vi "Drive Distance and Speed.vi"(4 "Minimum Speed To ramp to":dbl, 6 "Distance to Start Slowing Down At":dbl, 8 "Wanted Distance Right":dbl, 9 "Wanted Distance Left":dbl, 10 "Wanted Speed Right":dbl, 11 "Wanted Speed Left":dbl) -> (0 "Finished Driving":bool, 1 "Right Output Speed":dbl, 2 "Left Output Speed":dbl)   [LabVIEW 2016]
uses:
  Framework/Robot Global Data.vi
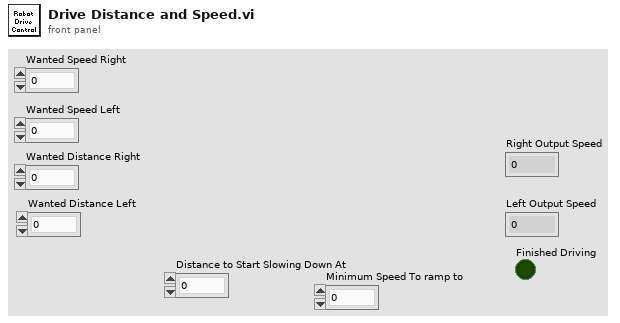
[diagram p1: front panel]
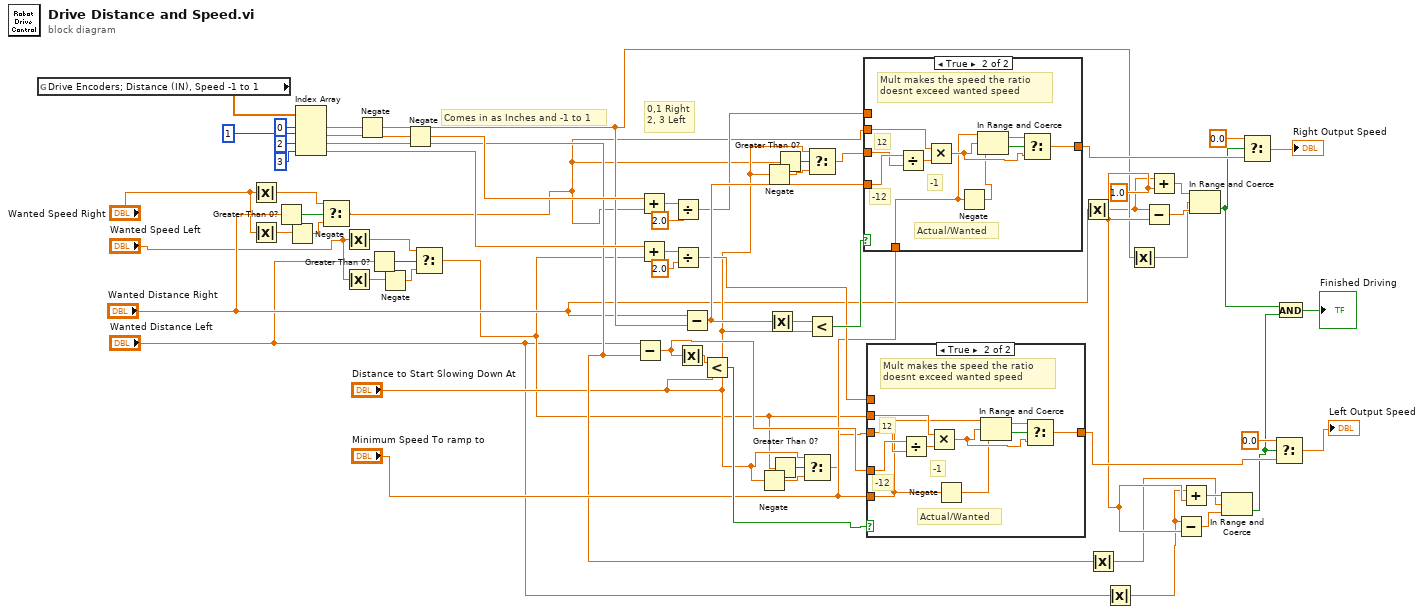
[diagram p0: block diagram]
diagram:
  w28 = 1.0 ("y")
  # "0,1 Right\n2, 3 Left"
  # "Comes in as Inches and -1 to 1"
  n1 = global read "Robot Global Data.vi" "Drive Encoders; Distance (IN), Speed -1 to 1"() -> (w63:dbl[])
  n2 = Absolute Value(x="Wanted Speed Right") -> (abs(x)=w15:dbl)
  n3 = Absolute Value(x="Wanted Speed Right") -> (abs(x)=w13:dbl)
  n4 = Greater Than 0?(x="Wanted Distance Right") -> (x > 0?=w17:bool)
  n5 = Negate(x=w13) -> (-x=w12:dbl)
  n6 = Index Array(array=w63, index #1=0 ("index"), index #2=1 ("index"), index #3=2 ("index"), index #4=3 ("index")) -> (element #1=w43:dbl, element #2=w60:dbl, element #3=w27:dbl, element #4=w58:dbl)
  n7 = Select(t=w15, s=w17, f=w12) -> (s? t:f=w18:dbl)
  n8 = Absolute Value(x="Wanted Speed Left") -> (abs(x)=w10:dbl)
  n9 = Absolute Value(x="Wanted Speed Left") -> (abs(x)=w9:dbl)
  n10 = Negate(x=w43) -> (-x=w26:dbl)
  n11 = Greater Than 0?(x="Wanted Distance Left") -> (x > 0?=w11:bool)
  n12 = Negate(x=w9) -> (-x=w8:dbl)
  n13 = Negate(x=w60) -> (-x=w33:dbl)
  n14 = Select(t=w10, s=w11, f=w8) -> (s? t:f=w7:dbl)
  n15 = Subtract(x="Wanted Distance Left", y=w27) -> (x-y=w51:dbl)
  n16 = Add(x=w33, y=w18) -> (x+y=w62:dbl)
  n17 = Add(x=w58, y=w7) -> (x+y=w59:dbl)
  n18 = Divide(x=w62, y=2.0) -> (x/y=w54:dbl)
  n19 = Divide(x=w59, y=2.0) -> (x/y=w50:dbl)
  n20 = Absolute Value(x=w51) -> (abs(x)=w49:dbl)
  n21 = Subtract(x="Wanted Distance Right", y=w26) -> (x-y=w55:dbl)
  n22 = Less?(x=w49, y="Distance to Start Slowing Down At") -> (x < y?=w52:bool)
  n23 = Negate(x="Distance to Start Slowing Down At") -> (-x=w20:dbl)
  n24 = Negate(x="Distance to Start Slowing Down At") -> (-x=w24:dbl)
  n25 = Absolute Value(x=w55) -> (abs(x)=w53:dbl)
  n26 = Greater Than 0?(x=w7) -> (x > 0?=w22:bool)
  n27 = Greater Than 0?(x=w18) -> (x > 0?=w23:bool)
  n28 = Select(t="Distance to Start Slowing Down At", s=w22, f=w20) -> (s? t:f=w19:dbl)
  n29 = Select(t="Distance to Start Slowing Down At", s=w23, f=w24) -> (s? t:f=w25:dbl)
  n30 = Less?(x=w53, y="Distance to Start Slowing Down At") -> (x < y?=w56:bool)
  n31 = case shown="True" w56 {
    tunnel: w25 -> [_ w73]
    tunnel: w55 -> [_ w74]
    tunnel: [w64 w72] -> w41
    tunnel: w54 -> [w64 _]
    tunnel: w18 -> [_ w70]
    tunnel: "Minimum Speed To ramp to" -> [_ w65]
    frame False {
    }
    frame True {
      # "12"
      # "-1"
      # "-12"
      # "Mult makes the speed the ratio doesnt exceed wanted speed"
      # "Actual/Wanted"
      n32 = Divide(x=w74, y=w73) -> (x/y=w71:dbl)
      n33 = Multiply(x=w70, y=w71) -> (x*y=w67:dbl)
      n34 = Negate(x=w65) -> (-x=w66:dbl)
      n35 = In Range and Coerce(upper limit=w65, x=w67, lower limit=w66) -> (coerced(x)=w68:dbl, In Range?=w69:bool)
      n36 = Select(t=w68, s=w69, f=w67) -> (s? t:f=w72:dbl)
    }
  }
  n37 = case shown="True" w52 {
    tunnel: w19 -> [_ w84]
    tunnel: w51 -> [_ w85]
    tunnel: [w75 w83] -> w37
    tunnel: w50 -> [w75 _]
    tunnel: w7 -> [_ w81]
    tunnel: "Minimum Speed To ramp to" -> [_ w76]
    frame False {
    }
    frame True {
      # "12"
      # "-1"
      # "-12"
      # "Mult makes the speed the ratio doesnt exceed wanted speed"
      # "Actual/Wanted"
      n38 = Divide(x=w85, y=w84) -> (x/y=w82:dbl)
      n39 = Multiply(x=w81, y=w82) -> (x*y=w78:dbl)
      n40 = Negate(x=w76) -> (-x=w77:dbl)
      n41 = In Range and Coerce(upper limit=w76, x=w78, lower limit=w77) -> (coerced(x)=w79:dbl, In Range?=w80:bool)
      n42 = Select(t=w79, s=w80, f=w78) -> (s? t:f=w83:dbl)
    }
  }
  n43 = Absolute Value(x="Wanted Distance Right") -> (abs(x)=w3:dbl)
  n44 = Absolute Value(x=w27) -> (abs(x)=w1:dbl)
  n45 = Absolute Value(x="Wanted Distance Left") -> (abs(x)=w2:dbl)
  n46 = Absolute Value(x=w26) -> (abs(x)=w4:dbl)
  n47 = Subtract(x=w3, y=w28) -> (x-y=w31:dbl)
  n48 = Add(x=w3, y=w28) -> (x+y=w32:dbl)
  n49 = Subtract(x=w2, y=w28) -> (x-y=w29:dbl)
  n50 = Add(x=w2, y=w28) -> (x+y=w30:dbl)
  n51 = In Range and Coerce(upper limit=w32, x=w4, lower limit=w31) -> (In Range?=w36:bool)  [unwired: 1 out]
  n52 = In Range and Coerce(upper limit=w30, x=w1, lower limit=w29) -> (In Range?=w35:bool)  [unwired: 1 out]
  n53 = Select(t=0.0, s=w36, f=w41) -> (s? t:f=→"Right Output Speed":dbl)
  n54 = Select(t=0.0, s=w35, f=w37) -> (s? t:f=→"Left Output Speed":dbl)
  n55 = And(x=w36, y=w35) -> (x .and. y?=→"Finished Driving":bool)
